vi "ex14-1.vi"   [LabVIEW 2014]
uses:
  <vilib>/NXT/Subs/MotorOutput.ctl
  <vilib>/NXT/Dual Mode Library/Motors/MotorDistance_Single.vi
types:
  T1 = typedef "MotorOutput.ctl" = u8
  T2 = typedef "LVHSConnector.ctl" = refnum<class "BrickReference.lvclass">
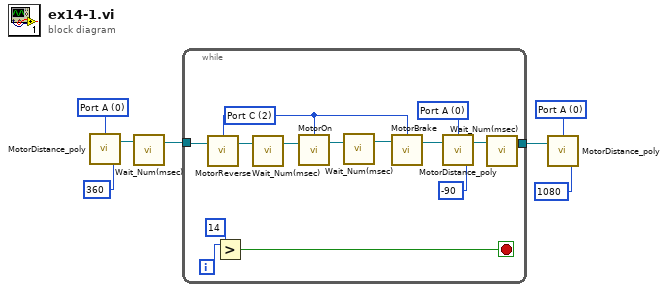
[diagram p0: block diagram]
diagram:
  w3 = T1 0 items=["Port A", "Port B", "Port C", "All Ports"] ("Output Port (All Ports)")
  w6 = T1 0 items=["Port A", "Port B", "Port C", "All Ports"] ("Output Port (All Ports)")
  n1 = call-poly <vilib>:"MotorDistance_poly.vi"("Angle of Rotation (360)"=360 ("Distance (100)"), "Output Port (All Ports)"=w6) -> ("NXT/EV3"=w5:T2)  [unwired: 2 in]
  n2 = call <vilib>:"Wait_Num(msec).vi"("NXT/EV3"=w5) -> ("NXT/EV3"=w4:T2)  [unwired: 3 in]
  n3 = while {
    tunnel: w4 -> [w14]
    tunnel: [w9] -> w1
    i -> [w21]
    stop <- w19 stop-if-true
    w12 = T1 0 items=["Port A", "Port B", "Port C", "All Ports"] ("Output Port (All Ports)")
    w8 = T1 2 items=["Port A", "Port B", "Port C", "All Ports"] ("Output Port (All Ports)")
    n4 = call <vilib>:"MotorReverse.vi"("NXT/EV3"=w14, "Output Port (All Ports)"=w8) -> ("NXT/EV3"=w17:T2)  [unwired: 2 in]
    n5 = Greater?(x=w21, y=14) -> (0:w19:bool)
    n6 = call <vilib>:"Wait_Num(msec).vi"("NXT/EV3"=w17) -> ("NXT/EV3"=w16:T2)  [unwired: 3 in]
    n7 = call <vilib>:"MotorOn.vi"("NXT/EV3"=w16, "Output Port (All Ports)"=w8) -> ("NXT/EV3"=w15:T2)  [unwired: 2 in]
    n8 = call <vilib>:"Wait_Num(msec).vi"("NXT/EV3"=w15) -> ("NXT/EV3"=w18:T2)  [unwired: 3 in]
    n9 = call <vilib>:"MotorBrake.vi"("NXT/EV3"=w18, "Port (All Ports)"=w8) -> ("NXT/EV3"=w10:T2)  [unwired: 2 in]
    n10 = call-poly <vilib>:"MotorDistance_poly.vi"("Angle of Rotation (360)"=-90 ("Distance (100)"), "NXT/EV3"=w10, "Output Port (All Ports)"=w12) -> ("NXT/EV3"=w13:T2)  [unwired: 1 in]
    n11 = call <vilib>:"Wait_Num(msec).vi"("NXT/EV3"=w13) -> ("NXT/EV3"=w9:T2)  [unwired: 3 in]
  }
  n12 = call-poly <vilib>:"MotorDistance_poly.vi"("Angle of Rotation (360)"=1080 ("Distance (100)"), "NXT/EV3"=w1, "Output Port (All Ports)"=w3) -> ()  [unwired: 1 in, 1 out]
